vi "BWC_analogSampleAveraged.vi"(11 "Acquisition Time (s)":dbl=1.0 caption="Acquisition Time (s) (no change)") -> (0 "Error Out":errorcluster, 1 "size(s)":i32=20001)   [LabVIEW 2017]
uses:
  <vilib>/Analysis/2dsp.llb/Power Spectrum (DBL).vi
  <vilib>/VirtualBench/_MSO Configure Analog Channel0.vi
  <vilib>/VirtualBench/_MSO Configure Timing8.vi
  <vilib>/Utility/file.llb/Write Delimited Spreadsheet (DBL).vi
  <vilib>/VirtualBench/VirtualBench.lvlib
  <vilib>/Analysis/NI_AALBase.lvlib
  <vilib>/Analysis/NI_AALPro.lvlib
panel:
  in  "write waveform":bool
  out "Analog Waveforms 2":waveform(dbl)(graph) caption="Analog Waveforms"
  in  "dark level":dbl
  out "(mean-darklvl)/std":dbl(graph)=0.019994885029411345
  out "std":dbl(graph)=0.019994885029411345
  out "mean-dark level":dbl(graph)=0.019994885029411345
  out "Analog Waveforms":waveform(dbl)[](graph)=[{"t0"=timestamp(3589833457.0102935 s since 1904-01-01), "dt"=5e-05, "Y"=array[20001 elements], "attributes"=variant("NI_ChannelName"=variant(string "mso/2"), "NI_UnitDescription"=variant(string "Volts"))}]
  in  "Auto Trigger":bool=TRUE caption="Auto Trigger (False)"
  in  "Pretrigger Time (s)":dbl=0.1 caption="Pretrigger Time (s) (no change)"
  in  "Sample Rate":dbl=20000.0 caption="Sample Rate (no change)"
  in  "Vertical Range":dbl=2.5 caption="Vertical Range (no change)"
  in  "Vertical Offset":dbl caption="Vertical Offset (no change)"
  in  "Probe Attenuation":i32(ring)=1 caption="Probe Attenuation (no change)" items=["1x"=1, "10x"=10]
  in  "Vertical Coupling":i32(ring)=1 caption="Vertical Coupling (no change)" items=["AC", "DC"]
  in  "Enable Channel":bool=TRUE caption="Enable Channel (no change)"
  in  "Channel":tag="mso/2"
  in  "Device Name":tag="VB8012-3059AE6"
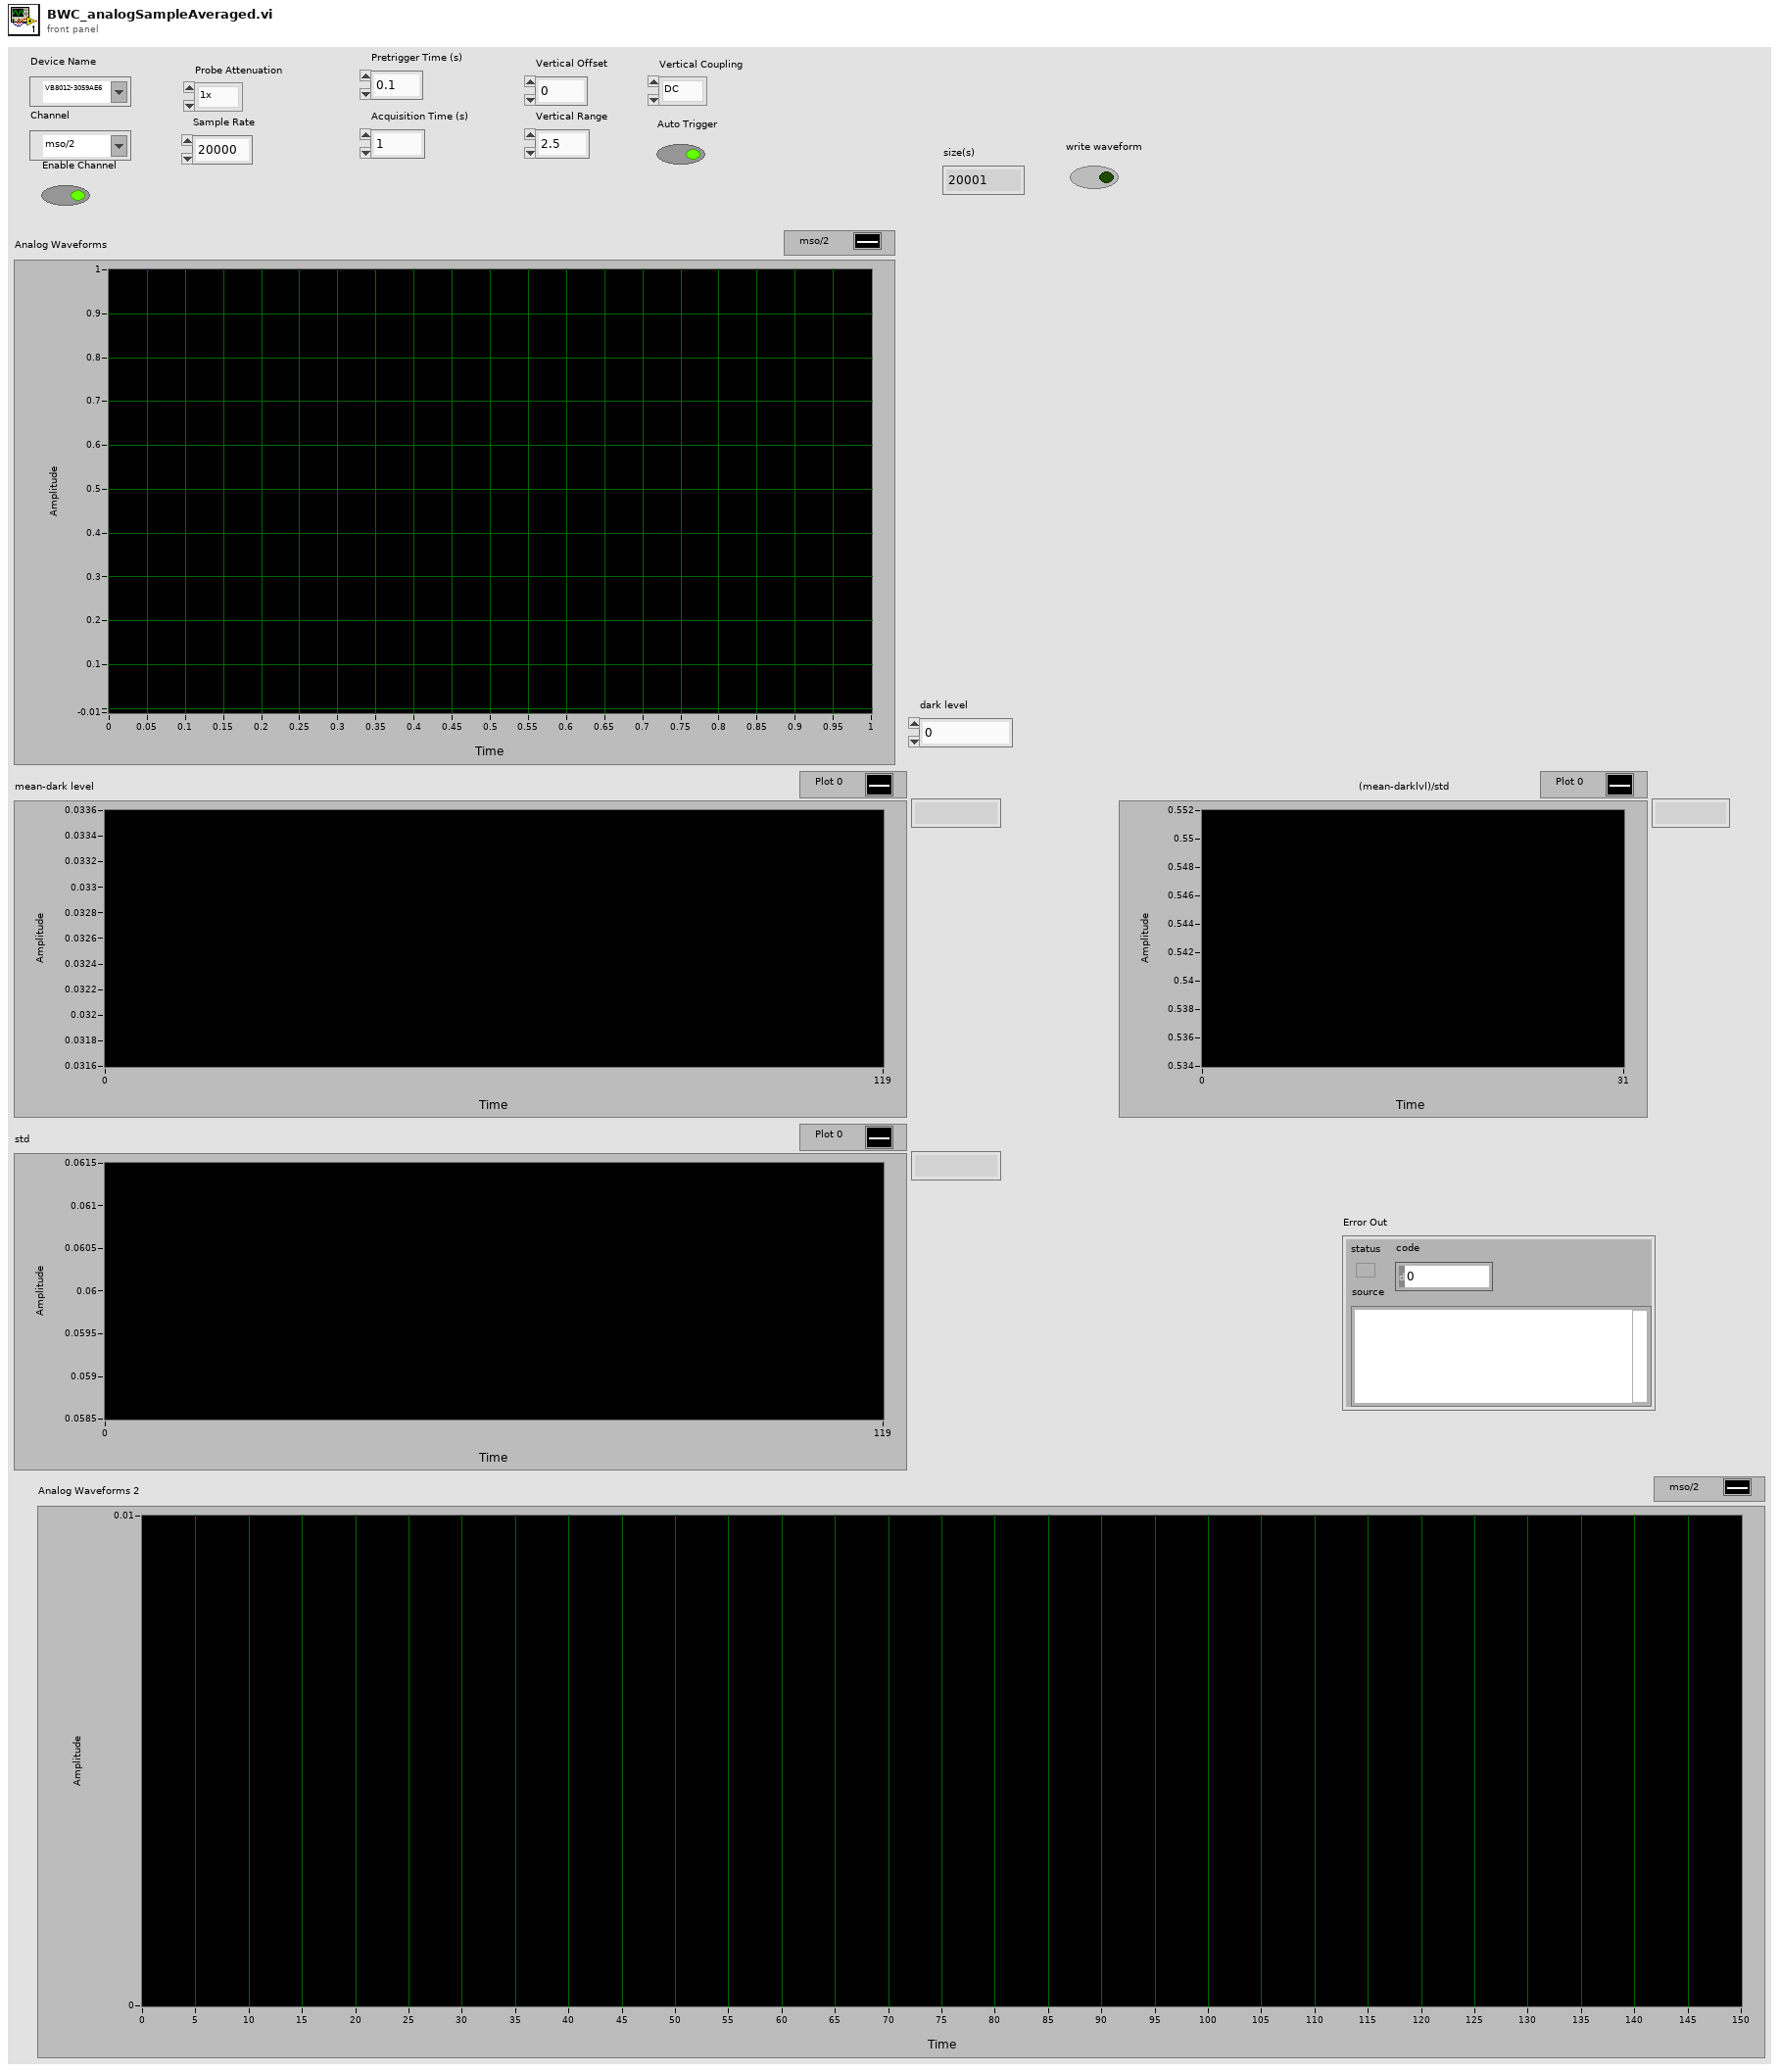
[diagram p1: front panel]
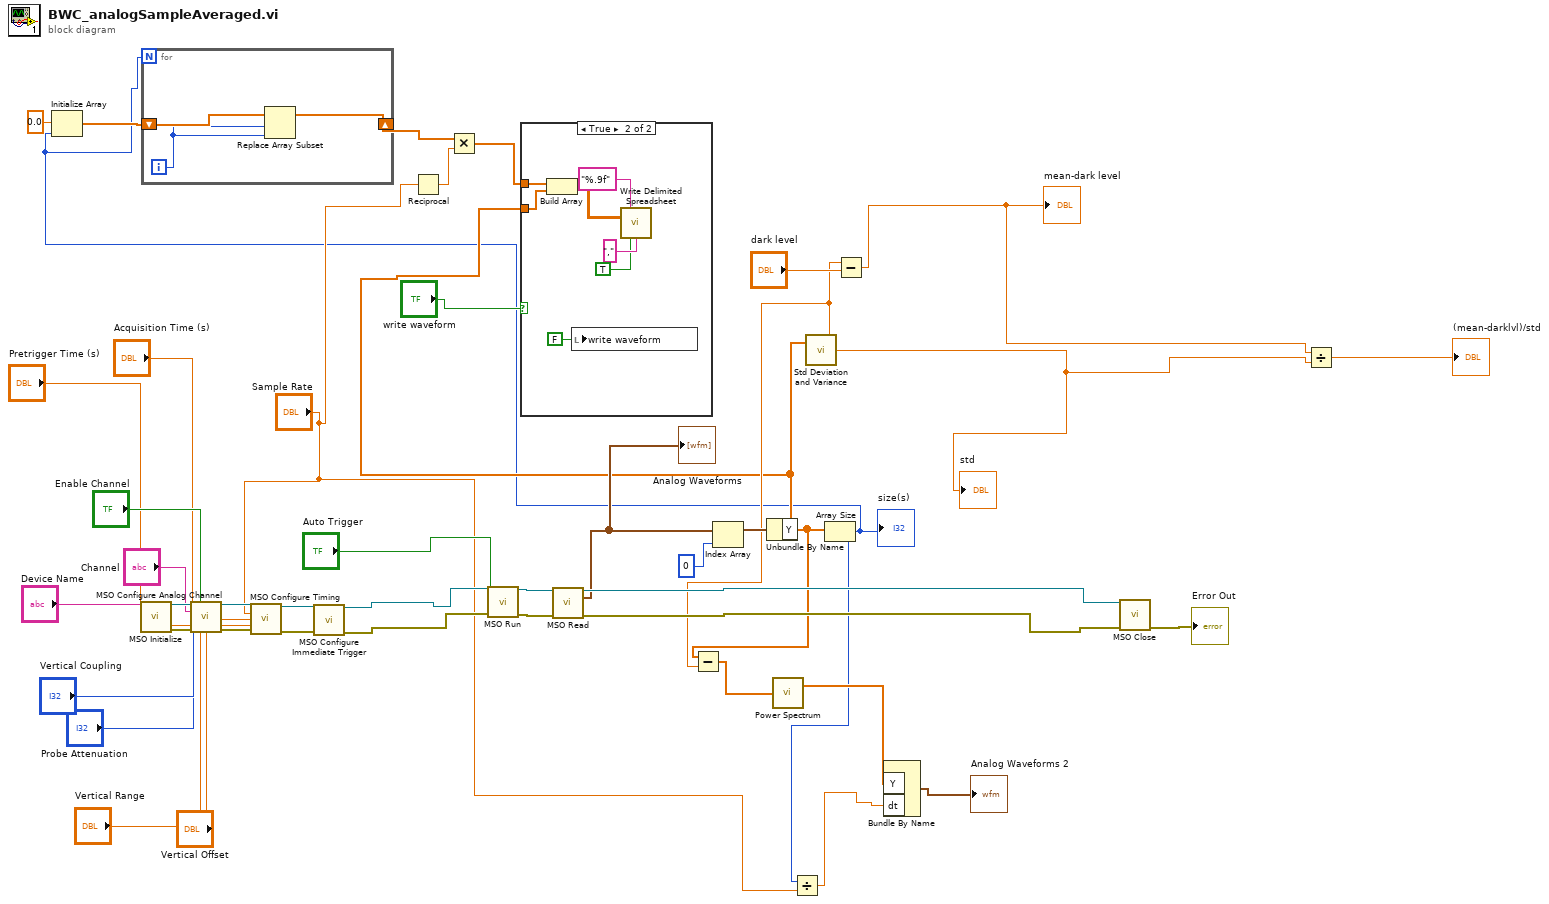
[diagram p0: block diagram]
diagram:
  n1 = call <vilib>:"MSO Initialize.vi"("Device Name"="Device Name") -> ("Instrument Handle Out"=w42:refnum<k21>, "Error Out"=w41:errorcluster)  [unwired: 13 in]
  n2 = call-poly <vilib>:"MSO Configure Analog Channel.vi"("Instrument Handle In"=w42, "Enable Channel"="Enable Channel", "Channel"="Channel", "Vertical Coupling"="Vertical Coupling", "Probe Attenuation"="Probe Attenuation", "Error In"=w41, "Vertical Range"="Vertical Range", "Vertical Offset"="Vertical Offset") -> ("Instrument Handle Out"=w39:refnum<k21>, "Error Out"=w37:errorcluster)  [unwired: 6 in]
  n3 = call-poly <vilib>:"MSO Configure Timing.vi"("Instrument Handle In"=w39, "Sample Rate"="Sample Rate", "Acquisition Time (s)"="Acquisition Time (s)", "Pretrigger Time (s)"="Pretrigger Time (s)", "Error In"=w37) -> ("Instrument Handle Out"=w38:refnum<k21>, "Error Out"=w36:errorcluster)  [unwired: 9 in]
  n4 = call <vilib>:"MSO Configure Immediate Trigger.vi"("Instrument Handle In"=w38, "Error In"=w36) -> ("Instrument Handle Out"=w23:refnum<k21>, "Error Out"=w24:errorcluster)  [unwired: 12 in]
  n5 = Reciprocal(x="Sample Rate") -> (1/x=w4:dbl)
  n6 = call <vilib>:"MSO Run.vi"("Instrument Handle In"=w23, "Auto Trigger"="Auto Trigger", "Error In"=w24) -> ("Instrument Handle Out"=w28:refnum<k21>, "Error Out"=w27:errorcluster)  [unwired: 11 in]
  n7 = call <vilib>:"MSO Read.vi"("Instrument Handle In"=w28, "Error In"=w27) -> ("Instrument Handle Out"=w20:refnum<k21>, "Analog Waveforms"=w9:waveform(dbl)[], "Error Out"=w21:errorcluster)  [unwired: 8 in, 3 out]
  "Analog Waveforms" <- w9
  n8 = Index Array(array=w9, index=0) -> (element=w25:waveform(dbl))
  n9 = Unbundle By Name(w25) -> ("Y"=w2:dbl[])
  n10 = call <vilib>:"Std Deviation and Variance.vi"("X"=w2) -> ("mean"=w14:dbl, "standard deviation"=w12:dbl)  [unwired: 1 in, 1 out]
  "std" <- w12
  n11 = Subtract(x=w2, y=w14) -> (x-y=w13:dbl[])
  n12 = call-poly <vilib>:"Power Spectrum.vi"("X"=w13) -> ("Power Spectrum"=w17:dbl[])  [unwired: 1 out]
  n13 = Array Size(array=w2) -> (size(s)=w1:i32)
  "size(s)" <- w1
  n14 = Initialize Array(0.0 ("element"), w1) -> (w7:dbl[])
  n15 = for {
    N: w1 -> [_]
    shift-right: [w45] -> w6
    shift-left: w7 -> [w47]
    i -> [w46]
    n16 = Replace Array Subset(array=w47, new element=w46, index=w46) -> (w45:dbl[])
  }
  n17 = Multiply(x=w6, y=w4) -> (x*y=w3:dbl[])
  n18 = case shown="True" "write waveform" {
    tunnel: w3 -> [_ w53]
    tunnel: w2 -> [_ w52]
    frame False {
    }
    frame True {
      n19 = Build Array(w53, w52) -> (w51:dbl[][])
      n20 = local write "write waveform"(FALSE ("write waveform")) -> ()
      n21 = call-poly <vilib>:"Write Delimited Spreadsheet.vi"("format (%.3f)"="%.9f", "2D data"=w51, "transpose? (no:F)"=TRUE, "delimiter (\\t)"="," ("delimiter (\\t)")) -> ()  [unwired: 10 in, 2 out]
    }
  }
  n22 = Divide(x=w1, y="Sample Rate") -> (x/y=w15:dbl)
  n23 = Subtract(x=w14, y="dark level") -> (x-y=w11:dbl)
  "mean-dark level" <- w11
  n24 = Bundle By Name("Y"=w17, "dt"=w15) -> (→"Analog Waveforms 2":waveform(dbl))  [unwired: 1 in]
  n25 = call <vilib>:"MSO Close.vi"("Instrument Handle In"=w20, "Error In"=w21) -> ("Error Out"=→"Error Out":errorcluster)  [unwired: 13 in]
  n26 = Divide(x=w11, y=w12) -> (x/y=→"(mean-darklvl)/std":dbl)
